vi "10_to_256.vi"(1 "Decimal":dbl format="%#_13g") -> (0 "256":u8[](array[numeric]))   [LabVIEW 2015, in "Igor.lvclass"]
uses:
  Igor.lvclass
panel:
  out "256 2":u8[](array[numeric])
  in  "Decimal 2":dbl format="%#_13g"
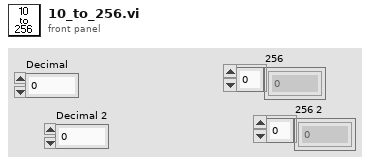
[diagram p1: front panel]
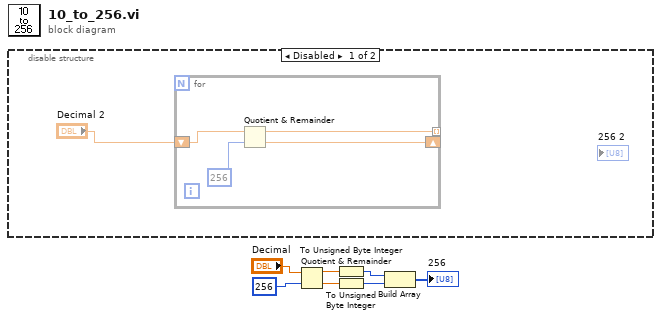
[diagram p0: block diagram]
diagram:
  n1 = disable-structure shown="Disabled" {
    frame Disabled {
      n2 = for {
        tunnel: [w10] -> _ mode=indexing
        shift-right: [w9] -> _
        shift-left: "Decimal 2" -> [w12]
        n3 = Quotient & Remainder(x=w12, y=256) -> (x-y*floor(x/y)=w10:dbl, floor(x/y)=w9:dbl)
      }
    }
    frame Enabled {
    }
  }
  n4 = Quotient & Remainder(x="Decimal", y=256) -> (x-y*floor(x/y)=w5:dbl, floor(x/y)=w4:dbl)
  n5 = To Unsigned Byte Integer(number=w5) -> (unsigned 8bit integer=w2:u8)
  n6 = To Unsigned Byte Integer(number=w4) -> (unsigned 8bit integer=w3:u8)
  n7 = Build Array(w2, w3) -> (→"256":u8[])
